vi "Draw_Path.vi"(1 "Group":string, 2 "PathM":dbl[][](array[numeric]), 3 "Image Out 2":T1) -> (0 "Image Out":T1)   [LabVIEW 2014]
doc: "根据路径坐标点在二维图中画线"
uses:
  <vilib>/vision/Image Controls.llb/IMAQ Image.ctl
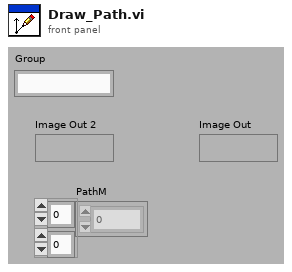
[diagram p1: front panel]
types:
  T1 = typedef "IMAQ Image.ctl" = refnum<image>
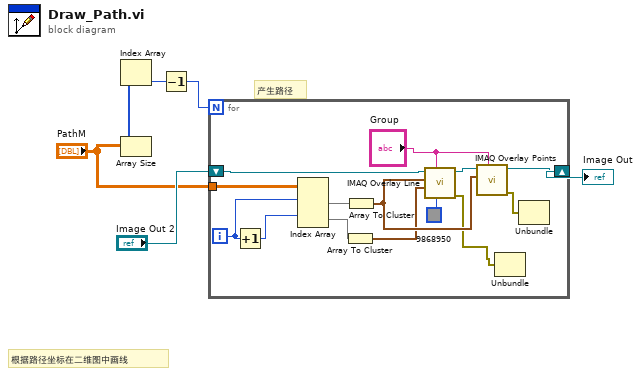
[diagram p0: block diagram]
diagram:
  # "根据路径坐标在二维图中画线"
  # "产生路径"
  n1 = Array Size(array="PathM") -> (size(s)=w1:i32[])
  n2 = Index Array(array=w1) -> (element=w3:i32)  [unwired: 1 in]
  n3 = Decrement(x=w3) -> (x-1=w2:i32)
  n4 = for {
    N: w2 -> [_]
    shift-right: [w16] -> w6
    shift-left: "Image Out 2" -> [w18]
    tunnel: "PathM" -> [w19]
    i -> [w15]
    n5 = Increment(x=w15) -> (x+1=w11:i32)
    n6 = Index Array(array=w19, index (row) #1=w15, index (row) #2=w11) -> (element #1=w20:dbl[], element #2=w10:dbl[])  [unwired: 2 in]
    n7 = Array To Cluster(array=w10) -> (cluster=w13:cluster{"PathM[0]":dbl, "PathM[1]":dbl})
    n8 = Array To Cluster(array=w20) -> (cluster=w14:cluster{"PathM[0]":dbl, "PathM[1]":dbl})
    n9 = call "IMAQ Overlay Line"("Color"=u32 9868950, "Group"="Group", "End Point"=w13, "Start Point"=w14, "Image"=w18) -> ("error out"=w8:errorcluster, "Image Out"=w17:T1)  [unwired: 5 in]
    n10 = call "IMAQ Overlay Points"("Group"="Group", "Point"=w14, "Image"=w17) -> ("error out"=w7:errorcluster, "Image Out"=w16:T1)  [unwired: 7 in]
    n11 = Unbundle(w8) -> ()  [unwired: 3 out]
    n12 = Unbundle(w7) -> ()  [unwired: 3 out]
  }
  "Image Out" <- w6
